vi "CD Init_Prepare Async Data_RT to BC and RT to RT.vi"(8 "error in (no error)":errorcluster, 10 "Card Parameters (in)":T1, 11 "Channels In":T8[](array[typedef]) {"RTs"."Mode Codes"."Words Item Refs" format="%.0x"; "RTs"."Mode Codes"."Timestamp Channel Data Reference" format="%.0x"; "RTs"."subAddresses"."Words Item Refs" format="%.0x"; "RTs"."subAddresses"."Timestamp Channel Data Reference" format="%.0x"; "RTs"."Status Channel Data Reference" format="%.0x"; "RTs"."Command Channels Refs" format="%.0x"; "BC"."Acyclic Frames Trigger Channels Refs" format="%.0x"; "BC"."Command Channels Refs" format="%.0x"; "BC"."messages"."Timestamp Channel Data Reference" format="%.0x"; "BC"."messages"."Status Channel Data Refs" format="%.0x"; "BC"."messages"."Words Item Refs" format="%.0x"; "BC"."messages"."Words Block Data Refs"."Data Reference" format="%.0x"}) -> (0 "error out":errorcluster, 2 "Raw Values (RT to BC)":T3, 3 "Map (RT to BC)":T5[](array[typedef]) {"Word Data Reference" format="%.0x"})   [LabVIEW 2017, in "Ballard MIL-1553 Engine.lvlib"]
doc: "This VI creates a static association between NI-VS FIFO Channel Index and Physical Channel, Label Index, Parameter Index for Parameter Channel of a Tx Scheduled Label."
uses:
  Ballard MIL-1553 Engine.lvlib
  Shared/Controls and Global/RT Channel.ctl
  Shared/Controls and Global/RT BC.ctl
  <vilib>/NI Veristand/Custom Device API/Custom Device Item Ref.ctl
  Shared/Controls and Global/RT Message.ctl
  Shared/Controls and Global/RT messageType.ctl
  Shared/Controls and Global/RT CWD1.ctl
  Shared/Controls and Global/RT CWD2.ctl
  <vilib>/NI Veristand/Custom Device API/Data Reference.ctl
  <vilib>/NI Veristand/Custom Device API/Block Data Reference.ctl
  Shared/Controls and Global/RT Remote Terminal.ctl
  Shared/Controls and Global/RT Remote Terminal_rtMode.ctl
  Shared/Controls and Global/RT Remote Terminal_RT subAddress.ctl
  Shared/Controls and Global/RT Remote Terminal_RT direction.ctl
  Shared/Controls and Global/RT Remote Terminal_RT Mode Code.ctl
  Controls/RT Async_Map RT2BC.ctl
  Controls/RT Async_Map_Type.ctl
  Controls/RT Async_Raw Values.ctl
  Controls/RT Async_Raw Values to Messages Index_Association.ctl
  Controls/Card Parameters.ctl
  Shared/Controls and Global/Initialization Method.ctl
  Controls/RT Async_Raw Values_Association.ctl
  <instrlib>/BTI1553Lib/Public/Controls/1553 RT Transfer Type.ctl
  <instrlib>/BTI1553Lib/Public/Controls/1553 Transfer Direction.ctl
  <instrlib>/BTI1553Lib/Private/RT/Configure/Get RT Xfer Handle.vi
  <vilib>/NI VeriStand/Custom Device API/Custom Device API.lvlib
  <instrlib>/BTI1553Lib/BTI1553LV.lvlib
  <vilib>/NI VeriStand/Custom Device Tools/Custom Device Utility Library/Custom Device Utility Library.lvlib
  Shared/Ballard 1553 Shared.lvlib
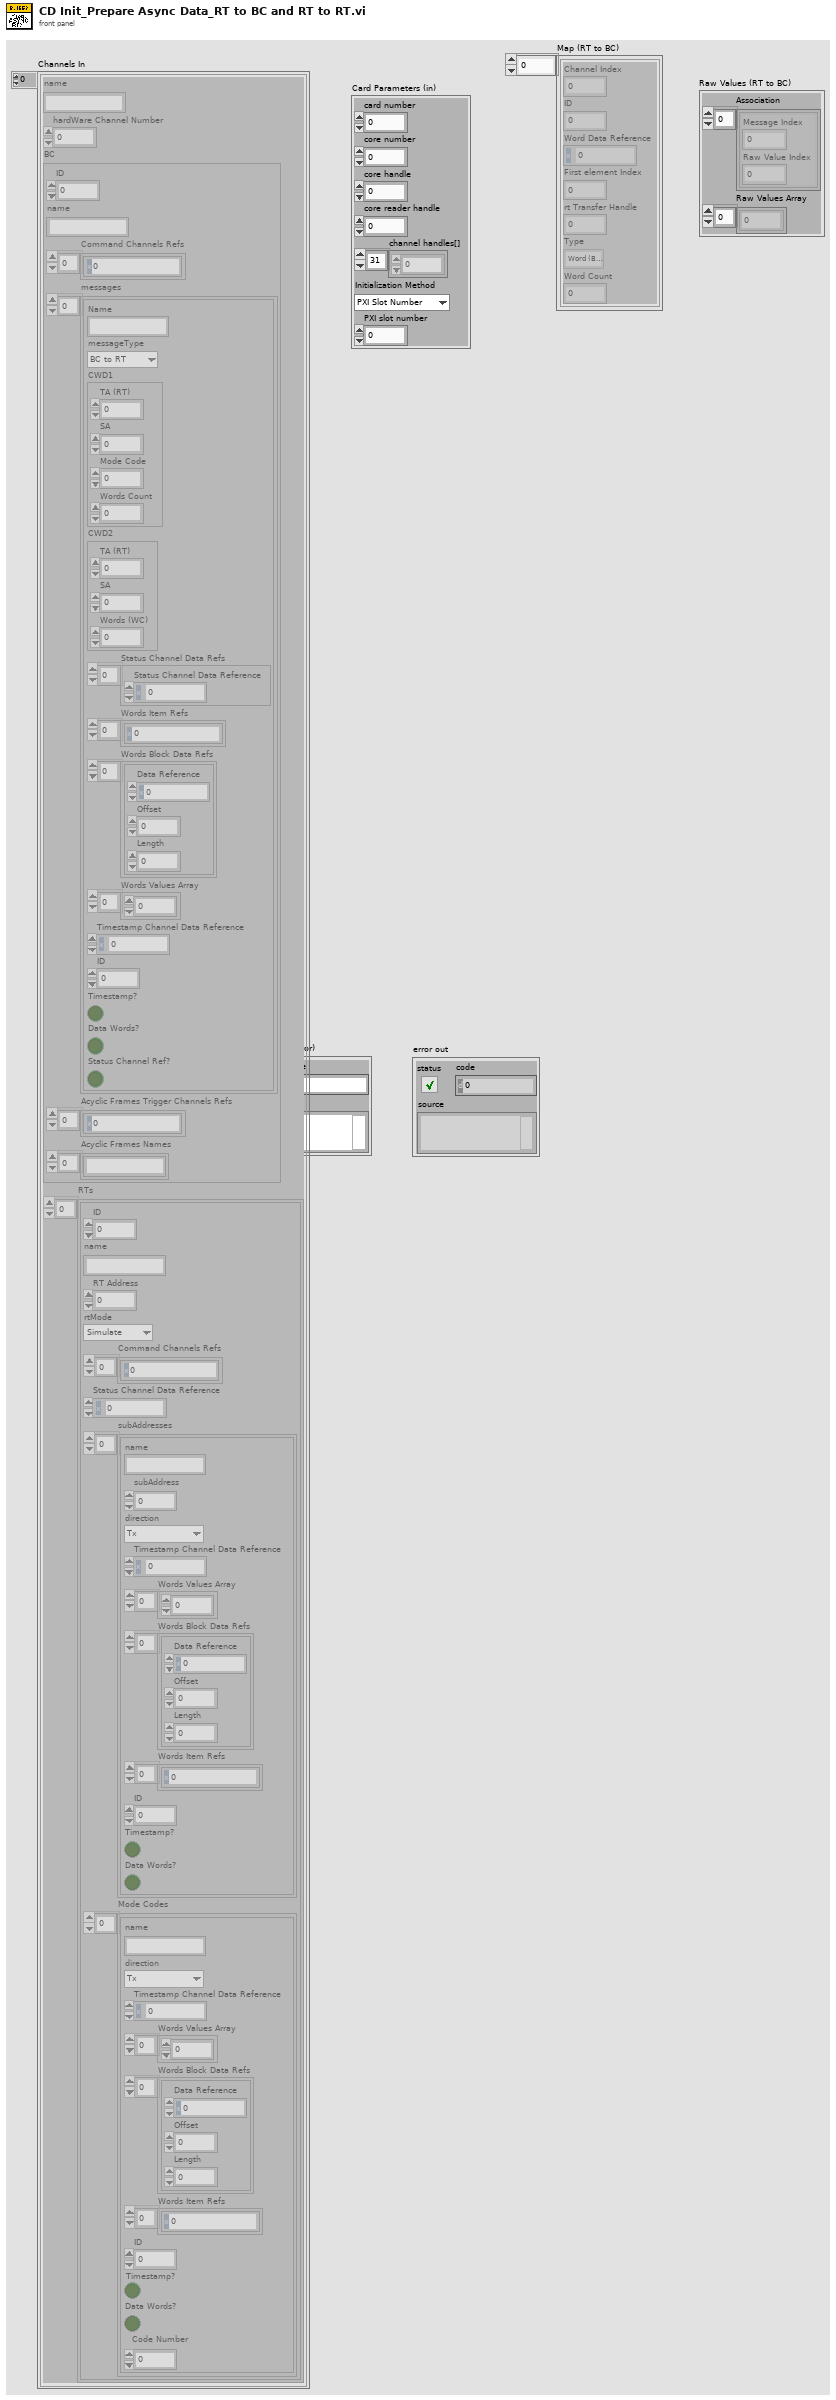
[diagram p1: front panel]
types:
  T1 = typedef "Ballard MIL-1553 Engine.lvlib/Card Parameters.ctl" = cluster{"card number":i32, "core number":i32, "core handle":u64, "core reader handle":u64, "channel handles[]":u64[], "Initialization Method":T2, "PXI slot number":i32}
  T2 = typedef "Ballard 1553 Shared.lvlib/Initialization Method.ctl" = enum16{"PXI Slot Number", "Card Number"}
  T3 = typedef "Ballard MIL-1553 Engine.lvlib/RT Async_Raw Values.ctl" = cluster{"Association":T4[], "Raw Values Array":u16[]}
  T4 = typedef "Ballard MIL-1553 Engine.lvlib/RT Async_Raw Values to Messages Index_Association.ctl" = cluster{"Message Index":i32, "Raw Value Index":i32}
  T5 = typedef "Ballard MIL-1553 Engine.lvlib/RT Async_Map RT2BC.ctl" = cluster{"Channel Index":i32, "ID":i32, "Word Data Reference":T6, "First element Index":i32, "rt Transfer Handle":u64, "Type":T7, "Word Count":i32}
  T6 = typedef "Custom Device API.lvlib/Data Reference.ctl" = i32
  T7 = typedef "Ballard MIL-1553 Engine.lvlib/RT Async_Map_Type.ctl" = enum16{"Word (BC to RT)", "Word (MC (Rx))", "Acyclic Message Trigger", "Word (RT to ..)", "Word (RT to RT)", "Word (MC (Tx))", "RT Status", "BC Commands", "RT Commands"}
  T8 = typedef "Ballard 1553 Shared.lvlib/RT Channel.ctl" = cluster{"name":string, "hardWare Channel Number":u16, "BC":T9, "RTs":T16[]}
  T9 = typedef "Ballard 1553 Shared.lvlib/RT BC.ctl" = cluster{"ID":i32, "name":string, "Command Channels Refs":T10[], "messages":T11[], "Acyclic Frames Trigger Channels Refs":T10[], "Acyclic Frames Names":string[]}
  T10 = typedef "Custom Device API.lvlib/Custom Device Item Ref.ctl" = u64
  T11 = typedef "Ballard 1553 Shared.lvlib/RT Message.ctl" = cluster{"Name":string, "messageType":T12, "CWD1":T13, "CWD2":T14, "Status Channel Data Refs":T6[], "Words Item Refs":T10[], "Words Block Data Refs":T15[], "Words Values Array":u16[], "Timestamp Channel Data Reference":T6, "ID":i32, "Timestamp?":bool, "Data Words?":bool, "Status Channel Ref?":bool}
  T12 = typedef "Ballard 1553 Shared.lvlib/RT messageType.ctl" = enum16{"BC to RT", "RT to BC", "RT to RT", "MC (Rx)", "MC (Tx)"}
  T13 = typedef "Ballard 1553 Shared.lvlib/RT CWD1.ctl" = cluster{"TA (RT)":i8, "SA":i8, "Mode Code":i8, "Words Count":i8}
  T14 = typedef "Ballard 1553 Shared.lvlib/RT CWD2.ctl" = cluster{"TA (RT)":i8, "SA":i8, "Words (WC)":i8}
  T15 = typedef "Custom Device API.lvlib/Block Data Reference.ctl" = cluster{"Data Reference":T6, "Offset":u64, "Length":u64}
  T16 = typedef "Ballard 1553 Shared.lvlib/RT Remote Terminal.ctl" = cluster{"ID":i32, "name":string, "RT Address":i32, "rtMode":T17, "Command Channels Refs":T10[], "Status Channel Data Reference":T6, "subAddresses":T18[], "Mode Codes":T20[]}
  T17 = typedef "Ballard 1553 Shared.lvlib/RT Remote Terminal_rtMode.ctl" = enum16{"Simulate", "Monitor", "Disable"}
  T18 = typedef "Ballard 1553 Shared.lvlib/RT Remote Terminal_RT subAddress.ctl" = cluster{"name":string, "subAddress":i8, "direction":T19, "Timestamp Channel Data Reference":T6, "Words Values Array":u16[], "Words Block Data Refs":T15[], "Words Item Refs":T10[], "ID":i32, "Timestamp?":bool, "Data Words?":bool}
  T19 = typedef "Ballard 1553 Shared.lvlib/RT Remote Terminal_RT direction.ctl" = enum16{"Tx", "Rx"}
  T20 = typedef "Ballard 1553 Shared.lvlib/RT Remote Terminal_RT Mode Code.ctl" = cluster{"name":string, "direction":T19, "Timestamp Channel Data Reference":T6, "Words Values Array":u16[], "Words Block Data Refs":T15[], "Words Item Refs":T10[], "ID":i32, "Timestamp?":bool, "Data Words?":bool, "Code Number":i32}
  T21 = typedef "Ballard MIL-1553 Engine.lvlib/RT Async_Raw Values_Association.ctl" = cluster{"Channel Data Reference":T6, "Raw Value Index":i32}
  T22 = typedef "BTI1553LV.lvlib/1553 Transfer Direction.ctl" = u32
  T23 = typedef "BTI1553LV.lvlib/1553 RT Transfer Type.ctl" = u32
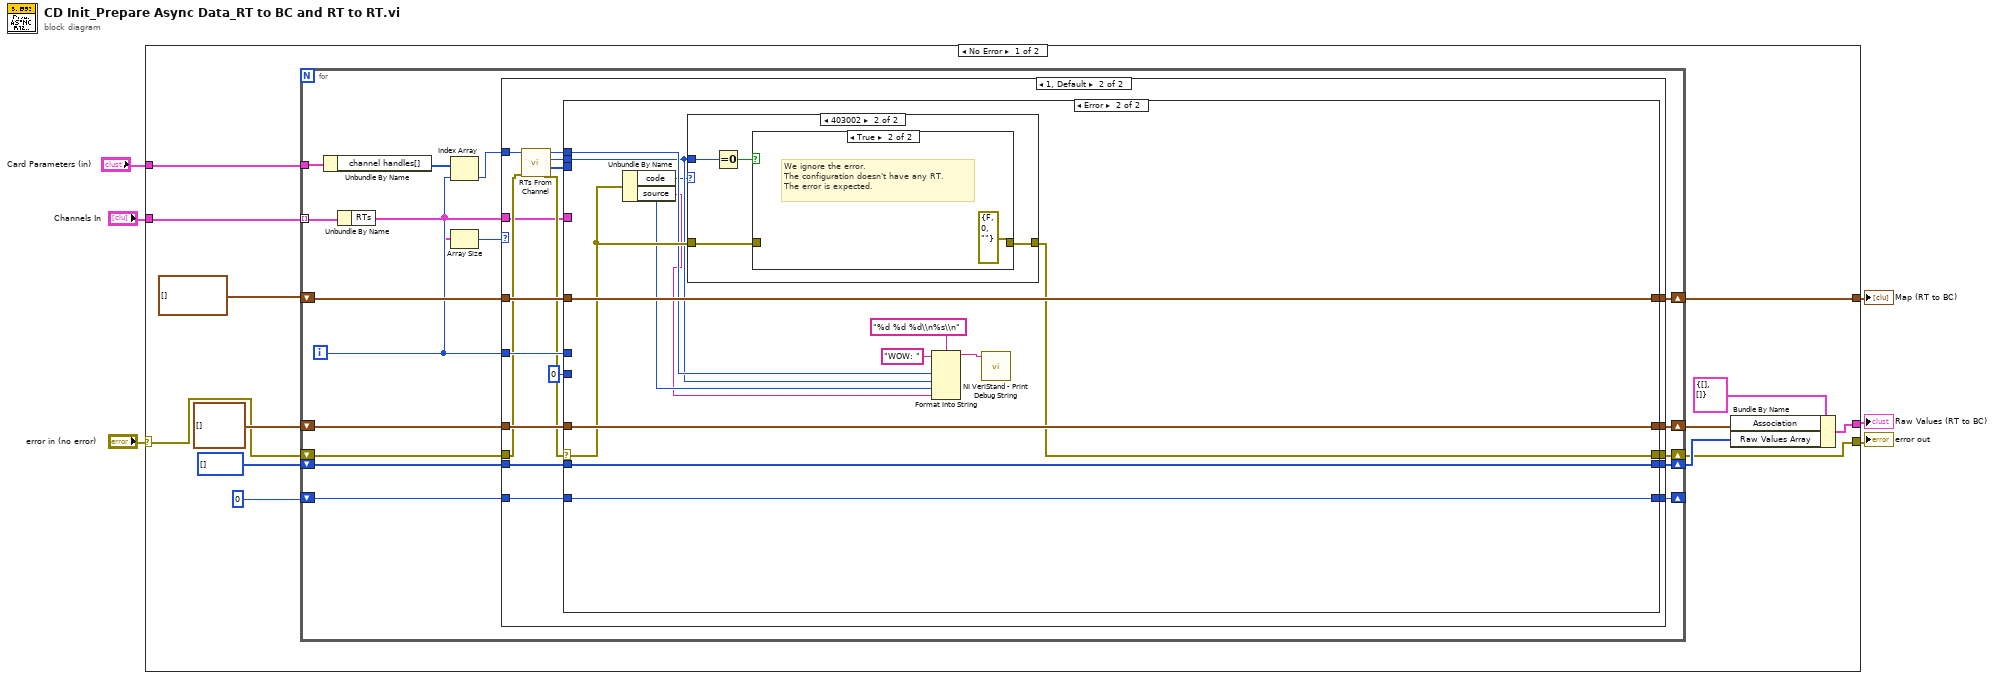
[diagram p0: block diagram]
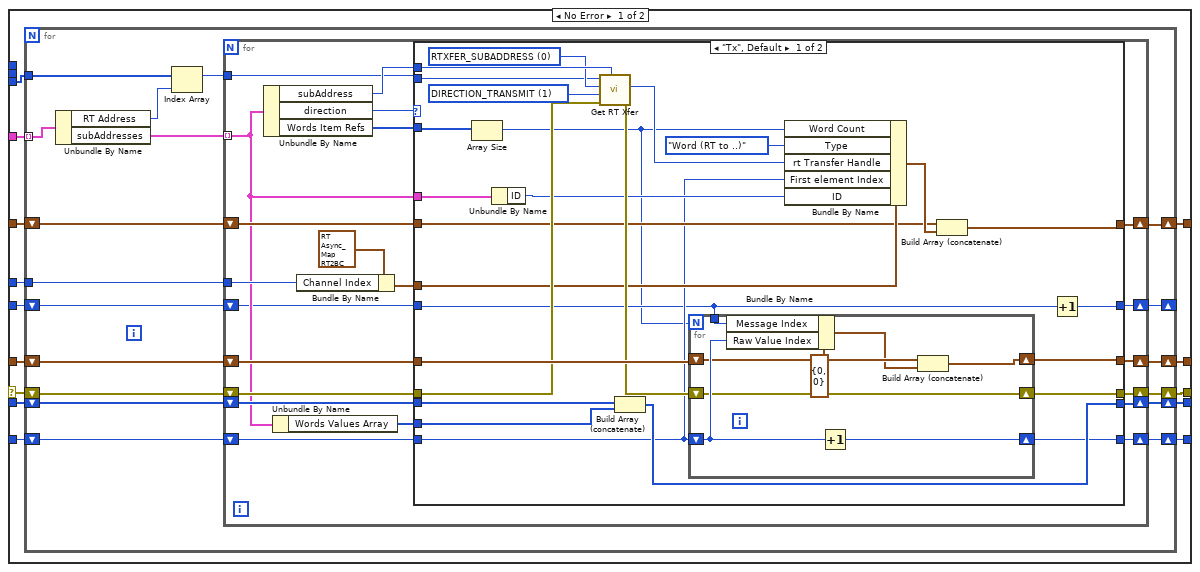
[diagram p3: hidden frame]
diagram:
  n1 = case shown="No Error" "error in (no error)" {
    selector: "error in (no error)" -> [w8 w173]
    tunnel: [w7 w173] -> w5
    tunnel: "Channels In" -> [w19 _]
    tunnel: [w17 _] -> w3
    tunnel: [w13 _] -> w2
    tunnel: "Card Parameters (in)" -> [w9 _]
    frame No Error {
      n2 = for {
        tunnel: w19 -> [w36] mode=indexing
        shift-right: [w34] -> w17
        shift-left: T5[] [] -> [w35]
        shift-right: [w32] -> w14
        shift-left: T21[] [] -> [w33]
        shift-right: [w28] -> w11
        shift-left: u16[] [] -> [w31]
        shift-right: [w29] -> _
        shift-left: 0 -> [w30]
        tunnel: w9 -> [w27]
        shift-right: [w24] -> w7
        shift-left: w8 -> [w23]
        i -> [w25]
        n3 = Unbundle By Name(w27) -> ("channel handles[]"=w26:u64[])
        n4 = Unbundle By Name(w36) -> ("RTs"=w21:T16[])
        n5 = Index Array(array=w26, index=w25) -> (element=w22:u64)
        n6 = Array Size(array=w21) -> (size(s)=w20:i32)
        n7 = case shown="1, Default" w20 {
          tunnel: w35 -> [w41 w59]
          tunnel: [w41 w58] -> w34
          tunnel: w33 -> [w40 w57]
          tunnel: [w40 w56] -> w32
          tunnel: w31 -> [w38 w55]
          tunnel: w30 -> [w37 w54]
          tunnel: [w37 w53] -> w29
          tunnel: [w38 w52] -> w28
          tunnel: w25 -> [_ w51]
          tunnel: [w39 w50] -> w24
          tunnel: w23 -> [w39 w49]
          tunnel: w22 -> [_ w44]
          tunnel: w21 -> [_ w43]
          frame 0 {
          }
          frame 1, Default {
            n8 = call <instrlib>:"RTs From Channel.vi"("error in (no error)"=w49, "channel handle in"=w44) -> ("error out"=w46:errorcluster, "remote terminal handles out"=w48:u64[], "remote terminal count out"=w45:i32, "channel handle out"=w42:u64)  [unwired: 6 in]
            n9 = case shown="Error" w46 {
              selector: w46 -> [w60 w161]
              tunnel: w43 -> [w73 _]
              tunnel: w59 -> [w72 w165]
              tunnel: [w71 w165] -> w58
              tunnel: w57 -> [w70 w164]
              tunnel: [w69 w164] -> w56
              tunnel: w55 -> [w68 w162]
              tunnel: w54 -> [w67 w163]
              tunnel: [w66 w163] -> w53
              tunnel: [w65 w162] -> w52
              tunnel: w51 -> [w64 _]
              tunnel: [w63 w160] -> w50
              tunnel: w48 -> [w62 _]
              tunnel: 0 -> [w61 _]
              tunnel: w45 -> [_ w157]
              tunnel: w42 -> [_ w158]
              frame No Error {
                n10 = for {
                  tunnel: w73 -> [w78] mode=indexing
                  shift-right: [w89] -> w71
                  shift-left: w72 -> [w90]
                  tunnel: w64 -> [w91]
                  shift-right: [w88] -> w69
                  shift-left: w70 -> [w84]
                  shift-right: [w87] -> w65
                  shift-left: w68 -> [w83]
                  shift-right: [w86] -> w66
                  shift-left: w67 -> [w85]
                  tunnel: w62 -> [w82]
                  shift-right: [w80] -> w63
                  shift-left: w60 -> [w81]
                  shift-right: [w74] -> _
                  shift-left: w61 -> [w75]
                  n11 = Unbundle By Name(w78) -> ("RT Address"=w76:i32, "subAddresses"=w79:T18[])
                  n12 = Index Array(array=w82, index=w76) -> (element=w77:u64)
                  n13 = for {
                    tunnel: w91 -> [w112]
                    tunnel: w79 -> [w95] mode=indexing
                    tunnel: w77 -> [w97]
                    shift-right: [w105] -> w86
                    shift-left: w85 -> [w104]
                    shift-right: [w99] -> w80
                    shift-left: w81 -> [w100]
                    shift-right: [w110] -> w89
                    shift-left: w90 -> [w111]
                    shift-right: [w107] -> w88
                    shift-left: w84 -> [w103]
                    shift-right: [w106] -> w87
                    shift-left: w83 -> [w102]
                    shift-right: [w92] -> w74
                    shift-left: w75 -> [w93]
                    n14 = Unbundle By Name(w95) -> ("subAddress"=w98:i8, "direction"=w94:T19, "Words Item Refs"=w108:T10[])
                    n15 = Unbundle By Name(w95) -> ("Words Values Array"=w101:u16[])
                    n16 = Bundle By Name(cluster=T5 {"Channel Index"=0, "ID"=0, "Word Data Reference"=0, "First element Index"=0, "rt Transfer Handle"=0, "Type"=enum."Word (BC to RT)", "Word Count"=0} ("Association"), "Channel Index"=w112) -> (w109:T5)
                    n17 = case shown="\"Tx\", Default" w94 {
                      tunnel: w111 -> [w119 w152]
                      tunnel: [w118 w152] -> w110
                      tunnel: w109 -> [w124 _]
                      tunnel: w108 -> [w116 _]
                      tunnel: [w125 w151] -> w107
                      tunnel: [w138 w149] -> w106
                      tunnel: [w137 w148] -> w105
                      tunnel: w104 -> [w115 w148]
                      tunnel: w103 -> [w136 w151]
                      tunnel: w102 -> [w135 w149]
                      tunnel: w101 -> [w134 _]
                      tunnel: w100 -> [w133 w150]
                      tunnel: [w131 w150] -> w99
                      tunnel: w98 -> [w130 _]
                      tunnel: w97 -> [w128 _]
                      tunnel: w95 -> [w127 _]
                      tunnel: w93 -> [w114 w147]
                      tunnel: [w117 w147] -> w92
                      frame "Tx", Default {
                        w126 = T22 1 items=["DIRECTION_RECEIVE", "DIRECTION_TRANSMIT"] ("transfer direction")
                        w129 = T23 0 items=["RTXFER_SUBADDRESS", "RTXFER_MODECODE"] ("transfer type")
                        n18 = Array Size(array=w116) -> (size(s)=w113:i32)
                        n19 = Unbundle By Name(w127) -> ("ID"=w121:i32)
                        n20 = call-poly <instrlib>:"Get RT Xfer.vi"("transfer sa number or mc number"=w130, "error in (no error)"=w133, "transfer direction"=w126, "transfer type"=w129, "remote terminal handle in"=w128) -> ("error out"=w132:errorcluster, "rt transfer handle out"=w122:u64)  [unwired: 4 in, 1 out]
                        n21 = Build Array (concatenate)(w135, w134) -> (w138:u16[])
                        n22 = for {
                          N: w113 -> [_]
                          shift-right: [w146] -> w137
                          shift-left: w115 -> [w145]
                          shift-right: [w143] -> w131
                          shift-left: w132 -> [w143]
                          shift-right: [w140] -> w125
                          shift-left: w136 -> [w144]
                          tunnel: w114 -> [w139]
                          n23 = Bundle By Name(cluster=T4 {"Message Index"=0, "Raw Value Index"=0}, "Message Index"=w139, "Raw Value Index"=w145) -> (w141:T4)
                          n24 = Increment(x=w145) -> (x+1=w146:i32)
                          n25 = Build Array (concatenate)(w144, w141) -> (w140:T21[])
                        }
                        n26 = Bundle By Name(cluster=w124, "Word Count"=w113, "Type"=RT_Async_Map_Type."Word (RT to ..)", "rt Transfer Handle"=w122, "First element Index"=w115, "ID"=w121) -> (w120:T5)
                        n27 = Build Array (concatenate)(w119, w120) -> (w118:T5[])
                        n28 = Increment(x=w114) -> (x+1=w117:i32)
                      }
                      frame "Rx" {
                      }
                    }
                  }
                }
              }
              frame Error {
                n29 = Unbundle By Name(w161) -> ("code"=w156:i32, "source"=w155:string)
                n30 = case shown="403002" w156 {
                  tunnel: w161 -> [w166 w168]
                  tunnel: w157 -> [_ w170]
                  tunnel: [w166 w167] -> w160
                  frame 0, Default {
                  }
                  frame 403002 {
                    n31 = Equal To 0?(x=w170) -> (x = 0?=w169:bool)
                    n32 = case shown="True" w169 {
                      tunnel: w168 -> [w171 _]
                      tunnel: [w171 errorcluster {"status"=FALSE, "code"=0, "source"=""} ("error IO")] -> w167
                      frame False {
                      }
                      frame True {
                        # "We ignore the error.\nThe configuration doesn't have any RT.\nThe error is expected."
                      }
                    }
                  }
                }
                n33 = Format Into String(format string="%d %d %d\\n%s\\n", initial string="WOW: ", w158, w157, w156, w155) -> (resulting string=w159:string)  [unwired: 1 in, 1 out]
                n34 = call <vilib>:"NI VeriStand - Print Debug String.vi"("Message"=w159) -> ()  [unwired: 10 in, 1 out]
              }
            }
          }
        }
      }
      n35 = Bundle By Name(cluster=T3 {"Association"=[], "Raw Values Array"=[]} ("Raw Values"), "Association"=w14, "Raw Values Array"=w11) -> (w13:T3)
    }
    frame Error {
    }
  }
  "error out" <- w5
  "Map (RT to BC)" <- w3
  "Raw Values (RT to BC)" <- w2
